vi "UHR-Fleezers Control (host) - 10.6.vi"() -> ()   [LabVIEW 2011] (continued)
        n2246 = call <vilib>:"Mean.vi"("X"=w3459) -> ("mean"=w3450:dbl)  [unwired: 1 out]
        n2247 = Subtract(x=w3554, y=w3546) -> (x-y=w3488:u64)
        n2248 = call <vilib>:"Mean.vi"("X"=w3544) -> ("mean"=w3485:dbl)  [unwired: 1 out]
        n2249 = Initialize Array(1.0 ("element"), w3453) -> (w3449:dbl[])
        n2250 = Initialize Array(1.0 ("element"), w3488) -> (w3479:dbl[])
        n2251 = Multiply(x=w3449, y=w3450) -> (x*y=w3451:dbl[])
        n2252 = Multiply(x=w3479, y=w3481) -> (x*y=w3482:dbl[])
        n2253 = Multiply(x=w3479, y=w3483) -> (x*y=w3484:dbl[])
        n2254 = Multiply(x=w3479, y=w3478) -> (x*y=w3480:dbl[])
        n2255 = Multiply(x=w3479, y=w3485) -> (x*y=w3486:dbl[])
        n2256 = Build Array (concatenate)(w3494, w3480) -> (w3548:dbl[])
        n2257 = Build Array (concatenate)(w3496, w3484) -> (w3552:dbl[])
        n2258 = Build Array (concatenate)(w3495, w3482) -> (w3551:dbl[])
        n2259 = Build Array (concatenate)(w3459, w3451) -> (w3461:dbl[])
        n2260 = Build Array (concatenate)(w3544, w3486) -> (w3553:dbl[])
        n2261 = Reshape Array(w3548, w3432, w3431) -> (w3514:dbl[][])
        n2262 = Reshape Array(w3461, w3432, w3431) -> (w3457:dbl[][])
        n2263 = Reshape Array(w3552, w3432, w3431) -> (w3506:dbl[][])
        n2264 = Reshape Array(w3551, w3432, w3431) -> (w3521:dbl[][])
        n2265 = Reshape Array(w3553, w3432, w3431) -> (w3531:dbl[][])
        n2266 = Array Subset(array=w3521, index (col)=0 ("index"), length (col)=w3446) -> (w3526:dbl[][])  [unwired: 2 in]
        n2267 = Array Subset(array=w3521, index (col)=w3446) -> (w3524:dbl[][])  [unwired: 3 in]
        n2268 = Array Subset(array=w3506, index (col)=0 ("index"), length (col)=w3446) -> (w3512:dbl[][])  [unwired: 2 in]
        n2269 = Array Subset(array=w3506, index (col)=w3446) -> (w3510:dbl[][])  [unwired: 3 in]
        n2270 = Array Subset(array=w3457, index (col)=0 ("index"), length (col)=w3446) -> (w3456:dbl[][])  [unwired: 2 in]
        n2271 = Array Subset(array=w3457, index (col)=w3446) -> (w3454:dbl[][])  [unwired: 3 in]
        n2272 = Array Subset(array=w3531, index (col)=0 ("index"), length (col)=w3446) -> (w3530:dbl[][])  [unwired: 2 in]
        n2273 = Array Subset(array=w3531, index (col)=w3446) -> (w3528:dbl[][])  [unwired: 3 in]
        n2274 = Array Subset(array=w3514, index (col)=0 ("index"), length (col)=w3446) -> (w3519:dbl[][])  [unwired: 2 in]
        n2275 = Array Subset(array=w3514, index (col)=w3446) -> (w3517:dbl[][])  [unwired: 3 in]
        n2276 = for {
          tunnel: w3526 -> [w3568] mode=indexing
          tunnel: [w3567] -> w3525 mode=indexing
          workers-P: _ -> [_]
          n2277 = Reverse 1D Array(array=w3568) -> (reversed array=w3567:dbl[])
        }
        n2278 = for {
          tunnel: w3512 -> [w3564] mode=indexing
          tunnel: [w3563] -> w3511 mode=indexing
          workers-P: _ -> [_]
          n2279 = Reverse 1D Array(array=w3564) -> (reversed array=w3563:dbl[])
        }
        n2280 = for {
          tunnel: w3456 -> [w3562] mode=indexing
          tunnel: [w3561] -> w3455 mode=indexing
          workers-P: _ -> [_]
          n2281 = Reverse 1D Array(array=w3562) -> (reversed array=w3561:dbl[])
        }
        n2282 = for {
          tunnel: w3530 -> [w3570] mode=indexing
          tunnel: [w3569] -> w3529 mode=indexing
          workers-P: _ -> [_]
          n2283 = Reverse 1D Array(array=w3570) -> (reversed array=w3569:dbl[])
        }
        n2284 = for {
          tunnel: w3519 -> [w3566] mode=indexing
          tunnel: [w3565] -> w3518 mode=indexing
          workers-P: _ -> [_]
          n2285 = Reverse 1D Array(array=w3566) -> (reversed array=w3565:dbl[])
        }
        n2286 = Index Array(array=w3531, index (row)=0) -> (element=→"Waveform Graph":dbl[])  [unwired: 1 in]
        n2287 = Add(x=w3525, y=w3524) -> (x+y=w3523:dbl[][])
        n2288 = Add(x=w3511, y=w3510) -> (x+y=w3509:dbl[][])
        n2289 = Add(x=w3455, y=w3454) -> (x+y=w3439:dbl[][])
        n2290 = Add(x=w3529, y=w3528) -> (x+y=w3503:dbl[][])
        n2291 = Add(x=w3518, y=w3517) -> (x+y=w3516:dbl[][])
        n2292 = Divide(x=w3509, y=2) -> (x/y=w3507:dbl[][])
        n2293 = Divide(x=w3523, y=2) -> (x/y=w3468:dbl[][])
        n2294 = Divide(x=w3516, y=2) -> (x/y=w3470:dbl[][])
        n2295 = To Single Precision Float(number=w3503) -> (single precision float=w3502:sgl[][])
        n2296 = Transpose 2D Array(2D array=w3507) -> (transposed array=→"Data map":dbl[][])
        n2297 = To Single Precision Float(number=w3439) -> (single precision float=w3443:sgl[][])
        n2298 = To Single Precision Float(number=w3468) -> (single precision float=w3474:sgl[][])
        n2299 = To Single Precision Float(number=w3470) -> (single precision float=w3471:sgl[][])
        n2300 = call "IMAQ ArrayToImage"("Image Pixels (Float)"=w3502, "Image"=w3436) -> ("Image Out"=w3505:T2)  [unwired: 8 in, 1 out]
        n2301 = call "IMAQ ArrayToImage"("Image Pixels (Float)"=w3443, "Image"=w3435) -> ("Image Out"=w3445:T2)  [unwired: 8 in, 1 out]
        n2302 = call "IMAQ ArrayToImage"("Image Pixels (Float)"=w3474, "Image"=w3434) -> ("Image Out"=w3476:T2)  [unwired: 8 in, 1 out]
        n2303 = call "IMAQ ArrayToImage"("Image Pixels (Float)"=w3471, "Image"=w3433) -> ("Image Out"=w3473:T2)  [unwired: 8 in, 1 out]
        n2304 = call "IMAQ Symmetry"("Type of Symmetry"=w3504, "Image Src"=w3505) -> ("Image Dst Out"=w3500:T2)  [unwired: 3 in, 1 out]
        n2305 = call "IMAQ Symmetry"("Type of Symmetry"=w3444, "Image Src"=w3445) -> ("Image Dst Out"=w3441:T2)  [unwired: 3 in, 1 out]
        n2306 = call "IMAQ Symmetry"("Type of Symmetry"=w3475, "Image Src"=w3476) -> ("Image Dst Out"=→"Detection Laser X":T2)  [unwired: 3 in, 1 out]
        n2307 = call "IMAQ Symmetry"("Type of Symmetry"=w3472, "Image Src"=w3473) -> ("Image Dst Out"=→"Detection Laser Y":T2)  [unwired: 3 in, 1 out]
        n2308 = call "IMAQ Set Simple Calibration"("Calibration Axis Info"=T35 {"Origin Pixel"={"X"=0.0, "Y"=0.0}, "Angle Relative to Horizontal (deg)"=0.0, "Axis Reference"=0}, "Grid Descriptor"=T36 {"X Step"=0.3, "Y Step"=0.3, "Unit"=enum."Undefined"}, "Image"=w3500) -> ("Calibrated Image"=→"APD 1":T2)  [unwired: 7 in, 1 out]
        n2309 = call "IMAQ Set Simple Calibration"("Calibration Axis Info"=T35 {"Origin Pixel"={"X"=0.0, "Y"=0.0}, "Angle Relative to Horizontal (deg)"=0.0, "Axis Reference"=0}, "Grid Descriptor"=T36 {"X Step"=0.3, "Y Step"=0.3, "Unit"=enum."Undefined"}, "Image"=w3441) -> ("Calibrated Image"=→"APD 2":T2)  [unwired: 7 in, 1 out]
      }
    }
    n2310 = Subtract(x=w2945, y="APD 2 Offset") -> (x-y=w2942:waveform(dbl))
    n2311 = Subtract(x=w2947, y="APD 1 Offset") -> (x-y=w2943:waveform(dbl))
    n2312 = Index Array(array=w2962, index=3) -> (element=w3022:waveform(dbl))
    n2313 = Index Array(array=w2962, index=6) -> (element=w3019:waveform(dbl))
    n2314 = Build Array(w2943, w2942) -> (→"APD Chart":waveform(dbl)[])
    n2315 = Array Size(array=w3013) -> (size(s)=w3066:i32)
    n2316 = call <vilib>:"Std Deviation and Variance.vi"("X"=w2955) -> ("standard deviation"=w2954:dbl)  [unwired: 1 in, 2 out]
    n2317 = Add Array Elements(numeric array=w2955) -> (sum=w2957:u32)
    n2318 = Add Array Elements(numeric array=w3013) -> (sum=w3076:u32)
    n2319 = call <vilib>:"Std Deviation and Variance.vi"("X"=w3013) -> ("standard deviation"=w3012:dbl)  [unwired: 1 in, 2 out]
    n2320 = Divide(x="T1 offset_x (mV)", y=1000.0) -> (x/y=w3023:dbl)
    n2321 = Divide(x=w2954, y=w2953) -> (x/y=w2950:dbl)
    "Rate sigma (Hz) 2" <- w2950
    n2322 = Multiply(x=w2953, y=w3066) -> (x*y=w2956:dbl)
    "Int. Time (s)" <- w2956
    n2323 = Divide(x=w2957, y=w2956) -> (x/y=w2951:dbl)
    "APD 2 Rate (Hz)" <- w2951
    n2324 = Divide(x=w3076, y=w2956) -> (x/y=w3010:dbl)
    "APD 1 Rate (Hz)" <- w3010
    n2325 = Divide(x=w3012, y=w2953) -> (x/y=w3011:dbl)
    "Rate sigma (Hz)" <- w3011
    n2326 = Divide(x=w2950, y=w2951) -> (x/y=→"Sigma/Mean 2":dbl)
    n2327 = Divide(x=w3011, y=w3010) -> (x/y=→"Sigma/Mean":dbl)
    n2328 = feedback-in #22("Calibration") -> ()
    n2329 = feedback #22(u16 1 ("Calibration")) -> (w3043:u16)
    n2330 = Divide(x="T2 offset_x (mV)", y=1000.0) -> (x/y=w3021:dbl)
    n2331 = case shown="0, Default" "Calibration" {
      tunnel: "T1 alpha_x (nm/V)" -> [_ w3399 w3420]
      tunnel: "T1 kappa_x (pN/nm)" -> [_ _ w3410]
      tunnel: "T2 alpha_x (nm/V)" -> [_ w3398 w3418]
      tunnel: "T2 kappa_x (pN/nm)" -> [_ _ w3411]
      tunnel: w3022 -> [w3381 w3396 w3416]
      tunnel: w3019 -> [w3380 w3394 w3414]
      tunnel: [w3381 w3393 w3413] -> w3052
      tunnel: [w3380 w3392 w3412] -> w3051
      tunnel: ["T1 X (V)" ("Label.Text") "T1 X (nm)" ("Label.Text") "T1 X (pN)" ("Label.Text")] -> w3040
      tunnel: ["T2 X (V)" ("Label.Text") "T2 X (nm)" ("Label.Text") "T2 X (pN)" ("Label.Text")] -> w3039
      tunnel: ["Position (V)" ("Label.Text") "Position (nm)" ("Label.Text") "Force (pN)" ("Label.Text")] -> w3041
      tunnel: w3021 -> [_ w3384 w3403]
      tunnel: w3023 -> [_ w3387 w3405]
      tunnel: ["Mean (V)" ("Label.Text") "Mean (nm)" ("Label.Text") "Mean (pN)" ("Label.Text")] -> w3036
      tunnel: ["Difference (V)" ("Label.Text") "Difference (nm)" ("Label.Text") "Difference (pN)" ("Label.Text")] -> w2970
      frame 0, Default {
      }
      frame 1 {
        n2332 = Unbundle By Name(w3396) -> ("Y"=w3400:dbl[])
        n2333 = Unbundle By Name(w3394) -> ("Y"=w3385:dbl[])
        n2334 = Subtract(x=w3400, y=w3387) -> (x-y=w3388:dbl[])
        n2335 = Subtract(x=w3385, y=w3384) -> (x-y=w3386:dbl[])
        n2336 = Multiply(x=w3386, y=w3398) -> (x*y=w3395:dbl[])
        n2337 = Multiply(x=w3399, y=w3388) -> (x*y=w3397:dbl[])
        n2338 = Bundle By Name(cluster=w3394, "Y"=w3395) -> (w3392:waveform(dbl))
        n2339 = Bundle By Name(cluster=w3396, "Y"=w3397) -> (w3393:waveform(dbl))
      }
      frame 2 {
        n2340 = Unbundle By Name(w3416) -> ("Y"=w3421:dbl[])
        n2341 = Unbundle By Name(w3414) -> ("Y"=w3419:dbl[])
        n2342 = Subtract(x=w3419, y=w3403) -> (x-y=w3404:dbl[])
        n2343 = Subtract(x=w3421, y=w3405) -> (x-y=w3406:dbl[])
        n2344 = Compound Arithmetic op=MULTIPLY(w3404, w3418, w3411) -> (w3415:dbl[])
        n2345 = Compound Arithmetic op=MULTIPLY(w3410, w3420, w3406) -> (w3417:dbl[])
        n2346 = Bundle By Name(cluster=w3414, "Y"=w3415) -> (w3412:waveform(dbl))
        n2347 = Bundle By Name(cluster=w3416, "Y"=w3417) -> (w3413:waveform(dbl))
      }
    }
    n2348 = Not Equal?(x=w3043, y="Calibration") -> (x != y?=w3000:bool)
    n2349 = case shown="True" w3000 {
      tunnel: w3041 -> [_ w3374]
      tunnel: w3040 -> [_ w3373]
      tunnel: w3039 -> [_ w3372]
      tunnel: w3036 -> [_ w3371]
      tunnel: w2970 -> [_ w3370]
      frame False {
      }
      frame True {
        n2350 = property on="Force" class="WFChart (strict)"("YScale.NameLbl.Text"=w3374) -> ()  [unwired: 2 in, 2 out]
        n2351 = property on="T2 X" class="DigNum (strict)"("Caption.Text"=w3372) -> ()  [unwired: 2 in, 2 out]
        n2352 = property on="T1 X" class="DigNum (strict)"("Caption.Text"=w3373) -> ()  [unwired: 2 in, 2 out]
        n2353 = property on="Mean" class="DigNum (strict)"("Caption.Text"=w3371) -> ()  [unwired: 2 in, 2 out]
        n2354 = property on="Difference" class="DigNum (strict)"("Caption.Text"=w3370) -> ()  [unwired: 2 in, 2 out]
      }
    }
    n2355 = Unbundle By Name(w3022) -> ("Y"=w3025:dbl[])
    n2356 = Unbundle By Name(w3019) -> ("Y"=w3028:dbl[])
    n2357 = Subtract(x=w3025, y=w3023) -> (x-y=w3026:dbl[])
    n2358 = Subtract(x=w3028, y=w3021) -> (x-y=w3027:dbl[])
    n2359 = Multiply(x=w3027, y="T2 alpha_x (nm/V)") -> (x*y=w2811:dbl[])
    n2360 = Multiply(x="T1 alpha_x (nm/V)", y=w3026) -> (x*y=w2812:dbl[])
    n2361 = Not(x="Trap Trig. Fl.") -> (.not. x?=w2849:bool)
    n2362 = Multiply(x=w3051, y=-1.0) -> (x*y=w3030:waveform(dbl))
    n2363 = Subtract(x=w2812, y=w2811) -> (x-y=w3018:dbl[])
    n2364 = Unbundle By Name(w3051) -> ("Y"=w2989:dbl[])
    n2365 = Unbundle By Name(w3052) -> ("Y"=w2813:dbl[])
    n2366 = Negate(x=w3018) -> (-x=w2809:dbl[])
    n2367 = Build Array(w3052, w3030) -> (→"Force":waveform(dbl)[])
    n2368 = Subtract(x=w2809, y="Offset (nm)") -> (x-y=w2987:dbl[])
    n2369 = case shown="True" "Read Lateness and Rel Phase" {
      tunnel: w2829 -> [w3347 w3369]
      tunnel: w2828 -> [w3348 w3368]
      tunnel: [w3347 w3367] -> w3016
      tunnel: [w3348 w3366] -> w3015
      frame False {
      }
      frame True {
        n2370 = xnode "Read/Write Control"("FPGA VI Reference In"=w3369, "error in"=w3368) -> ("FPGA VI Reference Out"=w3367:T19, "error out"=w3366:errorcluster, "GI Relative phase"=→"GI relative phase":i16, "Relative phase"=→"Relative phase (AI1)":i16, "AI Late Counter"=→"Late Counter (AI1)":u16, "GI Late Counter"=→"GI Late Counter":u16, "MCL Late Counter"=→"MCL Late Counter":u16, "MCL Relative Phase"=→"Relative Phase (MCL)":i16, "APD Acq Relative Phase"=→"APD Acq Relative Phase":i16, "APD 1 Gate Relative Phase"=→"APD 1 Gate Relative Phase":i16, "APD 2 Gate Relative Phase"=→"APD 2 Gate Relative Phase":i16, "APD Acq Late Counter"=→"APD Acq Late Counter":u16, "APD 1 Gate Late Counter"=→"APD 1 Gate Late Counter":u16, "APD 2 Gate Late Counter"=→"APD 2 Gate Late Counter":u16, "Green FB Relative Phase"=→"Relative phase (Green FB)":i16, "GI Relative phase 2"=→"GI relative phase 2":i16, "GI Late Counter 2"=→"GI Late Counter 2":u16, "Trap Pos FIFO Timeout"=→"Trap Pos FIFO Timeout":u16, "Trap AI FIFO Timeout"=→"Trap AI FIFO Timeout":u16)
      }
    }
    n2371 = call <vilib>:"Mean.vi"("X"=w2989) -> ("mean"=w2815:dbl)  [unwired: 1 out]
    "T2 X" <- w2815
    n2372 = Negate(x=w2989) -> (-x=w2990:dbl[])
    n2373 = call <vilib>:"Mean.vi"("X"=w2813) -> ("mean"=w2816:dbl)  [unwired: 1 out]
    "T1 X" <- w2816
    n2374 = Negate(x=w2815) -> (-x=w2814:dbl)
    n2375 = Bundle By Name(cluster=w3022, "Y"=w2987) -> (w2961:waveform(dbl))
    "Bead Separation" <- w2961
    n2376 = Add(x=w2813, y=w2990) -> (x+y=w2991:dbl[])
    n2377 = Add(x=w2816, y=w2814) -> (x+y=w3038:dbl)
    n2378 = Subtract(x=w2816, y=w2814) -> (x-y=→"Difference":dbl)
    n2379 = Divide(x=w2991, y=2.0) -> (x/y=→"Vec Mean of T1 T2":dbl[])
    n2380 = Divide(x=w3038, y=2.0) -> (x/y=w2993:dbl)
    "Mean" <- w2993
    n2381 = feedback-in #23("Trap Trig. Fl.") -> ()
    n2382 = feedback #23("Trap Trig. Fl.") -> (w2847:bool)
    n2383 = And(x=w2849, y=w2847) -> (x .and. y?=w2848:bool)
    n2384 = case "If have just turned off triggering" shown="True" w2848 {
      tunnel: w2829 -> [_ w3182]
      tunnel: w2828 -> [_ w3181]
      frame False {
      }
      frame True {
        w3180 = FALSE ("FPGA Trap Trig")
        n2385 = xnode "Read/Write Control"("FPGA VI Reference In"=w3182, "error in"=w3181, "FPGA Trap Trig"=w3180) -> ("FPGA VI Reference Out"=w3179:T19, "error out"=w3178:errorcluster)
        n2386 = xnode "Read/Write Control"("FPGA VI Reference In"=w3179, "error in"=w3178, "TTrig?"=w3180) -> ()  [unwired: 2 out]
        n2387 = local write "Initializing"(FALSE ("Initializing")) -> ()
        n2388 = local write "Triggered"(FALSE ("Triggered")) -> ()
        n2389 = local write "Waiting"(FALSE ("Waiting")) -> ()
      }
    }
    n2390 = Not(x=w2847) -> (.not. x?=w2860:bool)
    n2391 = And(x="Trap Trig. Fl.", y=w2860) -> (x .and. y?=w2857:bool)
    n2392 = local read "Tether"() -> (w2994:bool)
    n2393 = Or(x=w2857, y="Reinitialize") -> (x .or. y?=w2843:bool)
    n2394 = feedback #24(w2853) -> (w2858:string)
    n2395 = Select(t=w2853, s=w2857, f=w2858) -> (s? t:f=w2852:string)
    n2396 = Select(t=w2853, s="Reinitialize", f=w2852) -> (s? t:f=w2851:string)
    n2397 = feedback #25(0) -> (w2855:i32)
    n2398 = feedback #26(w2987) -> (w2986:dbl[])
    n2399 = Build Array (concatenate)(w2987, w2986) -> (w2810:dbl[])
    n2400 = case "For determining if there is a tether still" shown="True" w2994 {
      tunnel: w2993 -> [_ w3306]
      frame False {
      }
      frame True {
        n2401 = Greater?(x="Lost Tether Alarm Threshold (pN)", y=w3306) -> (0:w3304:bool)
        n2402 = case shown="True" w3304 {
          frame False {
          }
          frame True {
            w3307 = FALSE ("Value (Signaling)")
            n2403 = flat-sequence {
              frame #0 {
                # "stop only if saving"
                n2404 = local read "Saving..."() -> (w3319:bool)
                n2405 = And(x=w3319, y="TA Cancel Save?") -> (x .and. y?=w3318:bool)
                n2406 = local write "Stop Saving"(w3318) -> ()
              }
              frame #1 {
                n2407 = case shown="True" "TA Green Off?" {
                  frame False {
                  }
                  frame True {
                    w3322 = FALSE ("Fl. Triggered...")
                    n2408 = local write "Fl. Triggered..."(w3322) -> ()
                    n2409 = property on="Green Laser ON/Interlacing" class="Bool (strict)"("Val(Sgnl)"=w3322) -> ()  [unwired: 2 in, 2 out]
                  }
                }
              }
            }
            n2410 = local read "Time tether formed"() -> (w3313:timestamp)
            n2411 = Get Date/Time In Seconds() -> (seconds since 1Jan1904=w3314:timestamp)
            n2412 = Subtract(x=w3314, y=w3313) -> (x-y=w3312:dbl)
            n2413 = Number To Decimal String(number=w3312) -> (decimal integer string=w3309:string)  [unwired: 1 out]
            n2414 = local read "Messages"() -> (w3316:string)
            n2415 = call <vilib>:"Beep.vi"() -> ()  [unwired: 3 in, 9 out]
            n2416 = Concatenate Strings("Lost tether (" ("Message to add"), w3309, " s)." ("string")) -> (w3311:string)
            n2417 = local write "Tether"(FALSE ("Tether")) -> ()
            n2418 = call "Update messages.vi"("Message to add"=w3311, "Old message string"=w3316) -> ("New message string"=w3315:string)
            n2419 = local write "Messages"(w3315) -> ()
            n2420 = local write "Dip for Protein"(w3307) -> ()
            n2421 = property on="Trap Pos. FB ON" class="Bool (strict)"("Val(Sgnl)"=w3307) -> ()  [unwired: 2 in, 2 out]
            n2422 = property on="Trap Trig. Fl." class="Bool (strict)"("Val(Sgnl)"=w3307) -> ()  [unwired: 2 in, 2 out]
          }
        }
      }
    }
    n2423 = case "For triggering actions based on the trap position (e.g., turning the excitation laser on if trap under feedback moves so far)" shown="True" "Trap Trig. Fl." {
      tunnel: w2838 -> [_ w3195]
      tunnel: w2851 -> [_ w3194]
      tunnel: ["" ("t") w3193] -> w2859
      tunnel: w2843 -> [_ w3192]
      tunnel: [0 ("t") w3191] -> w2856
      tunnel: w2855 -> [_ w3190]
      tunnel: w2829 -> [_ w3189]
      tunnel: w2828 -> [_ w3188]
      frame False {
      }
      frame True {
        n2424 = case shown="\"Wait for trigger\"" w3194 {
          tunnel: w3195 -> [w3212 _ _ w3260]
          tunnel: [w3209 w3241 "" ("t") w3263] -> w3193
          tunnel: w3192 -> [_ _ _ w3251]
          tunnel: [w3208 w3238 0 ("t") w3252] -> w3191
          tunnel: w3190 -> [_ w3240 _ w3258]
          tunnel: w3189 -> [w3197 w3235 _ w3254]
          tunnel: w3188 -> [w3196 w3234 _ w3253]
          frame "Wait for trigger" {
            n2425 = local read "Trap Trig. (FPGA)"() -> (w3200:bool)
            n2426 = Subtract(x=w3212, y="Mean T1 Position\nto compare (nm)") -> (x-y=w3205:dbl[])
            n2427 = call <vilib>:"Std Deviation and Variance.vi"("X"=w3205) -> ("mean"=→"mean":dbl, "standard deviation"=→"standard\ndeviation":dbl)  [unwired: 1 in, 1 out]
            n2428 = Array Max & Min(array=w3205) -> (max value=→"max value":dbl, min value=→"min value":dbl)  [unwired: 2 out]
            n2429 = Greater?(x=w3205, y="Threshold (nm)") -> (0:w3215:bool[])
            n2430 = case shown="True" w3200 {
              tunnel: w3197 -> [_ w3221]
              tunnel: w3196 -> [_ w3220]
              tunnel: [FALSE ("TTrig?") w3219] -> w3203
              frame False {
              }
              frame True {
                n2431 = xnode "Read/Write Control"("FPGA VI Reference In"=w3221, "error in"=w3220) -> ("TTrig?"=w3219:bool)  [unwired: 2 out]
              }
            }
            n2432 = Or Array Elements(Boolean array=w3215) -> (logical OR=w3202:bool)
            n2433 = Select(t=w3203, s=w3200, f=w3202) -> (s? t:f=w3201:bool)
            n2434 = Not(x=w3200) -> (.not. x?=w3199:bool)
            n2435 = And(x=w3201, y=w3199) -> (x .and. y?=w3198:bool)
            n2436 = Select(t="Triggered", s=w3201, f="Wait for trigger") -> (s? t:f=w3209:string)
            n2437 = case shown="True" w3201 {
              tunnel: [0 0] -> w3208
              tunnel: w3197 -> [_ w3226]
              tunnel: w3196 -> [_ w3225]
              frame False {
                "Waiting" <- TRUE ("Waiting")
              }
              frame True {
                n2438 = xnode "Read/Write Control"("FPGA VI Reference In"=w3226, "error in"=w3225, "TTrig?"=FALSE) -> ()  [unwired: 2 out]
                n2439 = local read "Messages"() -> (w3229:string)
                n2440 = call <vilib>:"Beep.vi"() -> ()  [unwired: 12 in]
                n2441 = call "Update messages.vi"("Message to add"="Unwinding trigger.", "Old message string"=w3229) -> ("New message string"=w3230:string)
                n2442 = local write "Messages"(w3230) -> ()
                n2443 = local write "Waiting"(FALSE ("Waiting")) -> ()
                "Triggered" <- TRUE ("Triggered")
              }
            }
            n2444 = case "Only need to turn on laser if host triggered" shown="True" w3198 {
              frame False {
              }
              frame True {
                n2445 = property on="Green Laser ON/Interlacing" class="Bool (strict)"("Val(Sgnl)"=TRUE ("Value (Signaling)")) -> ()  [unwired: 2 in, 2 out]
              }
            }
          }
          frame "Triggered" {
            n2446 = local read "Trap Trig. (FPGA)"() -> (w3237:bool)
            n2447 = Increment(x=w3240) -> (x+1=w3238:i32)
            n2448 = Greater Or Equal?(x=w3238, y="Fl. ON time (n)") -> (x >= y?=w3236:bool)
            n2449 = Select(t="Wait for trigger", s=w3236, f="Triggered" ("t")) -> (s? t:f=w3241:string)
            n2450 = And(x=w3236, y=w3237) -> (x .and. y?=w3233:bool)
            n2451 = case shown="True" w3233 {
              tunnel: w3235 -> [_ w3245]
              tunnel: w3234 -> [_ w3244]
              frame False {
              }
              frame True {
                n2452 = xnode "Read/Write Control"("FPGA VI Reference In"=w3245, "error in"=w3244, "FPGA Trap Trig"=TRUE) -> ()  [unwired: 2 out]
              }
            }
            n2453 = case shown="True" w3236 {
              frame False {
              }
              frame True {
                w3247 = FALSE ("Value (Signaling)")
                n2454 = local write "Triggered"(w3247) -> ()
                n2455 = local write "Waiting"(TRUE ("Waiting")) -> ()
                n2456 = property on="Green Laser ON/Interlacing" class="Bool (strict)"("Val(Sgnl)"=w3247) -> ()  [unwired: 2 in, 2 out]
              }
            }
          }
          frame "Do nothing" {
          }
          frame "Initialize", Default {
            n2457 = Increment(x=w3258) -> (x+1=w3262:i32)
            n2458 = Select(t=1, s=w3251, f=w3262) -> (s? t:f=w3252:i32)
            n2459 = feedback #27(w3260) -> (w3266:dbl[])
            n2460 = Build Array (concatenate)(w3260, w3266) -> (w3259:dbl[])
            n2461 = Greater Or Equal?(x=w3252, y="Wait to get offset (n)") -> (x >= y?=w3255:bool)
            n2462 = Select(t=w3260, s=w3251, f=w3259) -> (s? t:f=w3261:dbl[])
            n2463 = feedback-in #27(w3261) -> ()
            n2464 = call <vilib>:"Mean.vi"("X"=w3261) -> ("mean"=w3256:dbl)  [unwired: 1 out]
            n2465 = local write "Mean T1 Position\nto compare (nm)"(w3256) -> ()
            n2466 = case shown="True" w3251 {
              tunnel: w3254 -> [_ w3272]
              tunnel: w3253 -> [_ w3271]
              frame False {
              }
              frame True {
                w3268 = FALSE ("FPGA Trap Trig")
                n2467 = xnode "Read/Write Control"("FPGA VI Reference In"=w3272, "error in"=w3271, "FPGA Trap Trig"=w3268) -> ("FPGA VI Reference Out"=w3270:T19, "error out"=w3269:errorcluster)
                n2468 = xnode "Read/Write Control"("FPGA VI Reference In"=w3270, "error in"=w3269, "TTrig?"=w3268) -> ()  [unwired: 2 out]
              }
            }
            n2469 = Select(t="Wait for trigger", s=w3255, f="Initialize") -> (s? t:f=w3263:string)
            n2470 = case shown="True" w3255 {
              tunnel: w3256 -> [_ w3275]
              tunnel: w3254 -> [_ w3284]
              tunnel: w3253 -> [_ w3283]
              frame False {
                n2471 = local write "Waiting"(FALSE ("Waiting")) -> ()
                "Initializing" <- TRUE ("Initializing")
              }
              frame True {
                n2472 = local read "Threshold (nm)"() -> (w3287:dbl)
                n2473 = local read "AOM X Cal (nm/MHz)"() -> (w3286:dbl)
                n2474 = Add(x=w3275, y=w3287) -> (x+y=w3288:dbl)
                n2475 = Divide(x=w3288, y=w3286) -> (x/y=w3285:dbl)
                n2476 = call "IR AOM freq to word.vi"("Frequency In (MHz)"=w3285) -> ("Frequency Word Out (double)"=w3282:dbl)
                n2477 = local write "Initializing"(FALSE ("Initializing")) -> ()
                n2478 = local write "Waiting"(TRUE ("Waiting")) -> ()
                n2479 = To Quad Integer(1:w3282) -> (0:w3281:i64)
                n2480 = xnode "Read/Write Control"("FPGA VI Reference In"=w3284, "error in"=w3283, "FPGA TTrig Thresh"=w3281) -> ("FPGA VI Reference Out"=w3278:T19, "error out"=w3277:errorcluster)
                n2481 = xnode "Read/Write Control"("FPGA VI Reference In"=w3278, "error in"=w3277, "FPGA Trap Trig"=TRUE) -> ()  [unwired: 2 out]
              }
            }
          }
        }
      }
    }
    n2482 = feedback-in #24(w2859) -> ()
    n2483 = feedback-in #25(w2856) -> ()
    n2484 = Split 1D Array(array=w2810, index=w2873) -> (first subarray=w2983:dbl[])  [unwired: 1 out]
    n2485 = feedback-in #26(w2983) -> ()
    n2486 = call <vilib>:"Mean.vi"("X"=w2983) -> ("mean"=w2982:dbl)  [unwired: 1 out]
    "Bead Mean (nm)" <- w2982
    n2487 = Subtract(x=w2983, y=w2982) -> (x-y=w2981:dbl[])
    n2488 = Square(x=w2981) -> (x^2=w2980:dbl[])
    n2489 = call <vilib>:"Mean.vi"("X"=w2980) -> ("mean"=w2979:dbl)  [unwired: 1 out]
    n2490 = Square Root(x=w2979) -> (sqrt(x)=w2978:dbl)
    n2491 = Multiply(x=10.0, y=w2978) -> (x*y=→"RMS (Ang)":dbl)
    n2492 = xnode "Read/Write Control"("FPGA VI Reference In"=w3016, "error in"=w3015) -> ("FPGA VI Reference Out"=w2841:T19, "error out"=w2840:errorcluster, "AI2 Y Sum Set 1"=w3122:i16, "AI2 Y Sum Set 2"=w3121:i16, "AI1 X Set 1"=w2905:fxp<+/-,16,1>, "AI1 X Set 2"=w2904:fxp<+/-,16,1>, "Trap Pos FB Int Signal"=→"Trap Pos FB Int Signal":fxp<+/-,24,9>, "Trap Pos FB Int-Norm Signal"=→"Trap Pos FB Int-Norm Signal":fxp<+/-,16,1>, "Trap Pos FB Action"=w2898:i64, "Scanning"=→"AOD Scanning":bool, "Scan I"=→"AOD Scan I":u64, "Scanning MCL"=w3124:bool, "Scan I (MCL)"=→"MCL Scan I":u64, "Green FB Signals"=w3061:T46, "TTrig Sig"=w2827:i64, "TTrig Fin Thresh"=w2823:i64)
    "MCL Scanning" <- w3124
    "Trap Pos FB Action" <- w2898
    n2493 = local read "FB Trig Integrate"() -> (w2821:u32)
    n2494 = Divide(x=w2827, y=w2821) -> (x/y=w2820:dbl)
    "TTrig Sig (Int)" <- w2820
    n2495 = Divide(x=w2823, y=w2821) -> (x/y=w2818:dbl)
    "TTrig Fin Thresh (Int)" <- w2818
    n2496 = local read "AOM X Cal (nm/MHz)"() -> (w2826:dbl)
    n2497 = local read "AI2 (V)"() -> (w3123:cluster{"Set 1":dbl, "Set 2":dbl})
    n2498 = Bundle By Name(cluster=w3123, "Set 1"=w3122, "Set 2"=w3121) -> (w3119:cluster{"Set 1":dbl, "Set 2":dbl})
    n2499 = Divide(x=w2898, y=327.67) -> (x/y=→"Action (%)":dbl)
    n2500 = local read "Trap X (AI1)"() -> (w2918:T10)
    n2501 = call "IR AOM word double to freq.vi"("Frequency Word In (double)"=w2818) -> ("Frequency Out (MHz)"=w2817:dbl)
    n2502 = call "IR AOM word double to freq.vi"("Frequency Word In (double)"=w2820) -> ("Frequency Out (MHz)"=w2819:dbl)
    n2503 = Divide(x=w3119, y=3276.7) -> (x/y=w3118:cluster{"Set 1":dbl, "Set 2":dbl})
    n2504 = Multiply(x=w2819, y=w2826) -> (x*y=w2825:dbl)
    "TTrig Sig (nm)" <- w2825
    n2505 = Multiply(x=w2817, y=w2826) -> (x*y=w2824:dbl)
    "TTrig Fin Thresh (nm)" <- w2824
    n2506 = local write "AI2 (V)"(w3118) -> ()
    n2507 = Bundle(cluster=w2918, "Trap 1"=w2905, "Trap 2"=w2904) -> (→"Trap X (AI1)":T10)
    n2508 = Bundle(w2825, w2824) -> (→"TTrig":cluster{dbl, dbl})  [unwired: 1 in]
    n2509 = Divide(x=w3061, y=3276.7) -> (x/y=w3057:T47)
    n2510 = Unbundle By Name(w3057) -> ("Green FB Ch 0"=w3060:dbl, "Green FB Ch 1"=w3059:dbl, "Green FB Ch 2"=w3058:dbl)
    n2511 = Divide(x=w3060, y=w3058) -> (x/y=w3056:dbl)
    n2512 = Divide(x=w3059, y=w3058) -> (x/y=w3055:dbl)
    n2513 = flat-sequence "To save data" {
      tunnel: [w4143] -> w3142
      tunnel: [w4144] -> w3141
      tunnel: w3092 -> [w4137]
      tunnel: w2846 -> [w4141]
      tunnel: ["Save Calibration"] -> w3115
      tunnel: w3112 -> [w4140]
      tunnel: [w4133] -> w3111
      tunnel: [w4130] -> w3110
      tunnel: [w4127] -> w3109
      tunnel: w3091 -> [w4129]
      tunnel: w2998 -> [w4123]
      tunnel: [w4123] -> w2997
      tunnel: ["Start Saving"] -> w2963
      tunnel: [w4117] -> w2886
      tunnel: [w4116] -> w2885
      tunnel: w3142 -> [w4378]
      tunnel: w3141 -> [w4377]
      tunnel: w2887 -> [w4376]
      tunnel: w3115 -> [w4375]
      tunnel: w3111 -> [w4373]
      tunnel: w3110 -> [w4372]
      tunnel: w3109 -> [w4371]
      tunnel: w2972 -> [w4370]
      tunnel: w3008 -> [w4369]
      tunnel: w2997 -> [w4368]
      tunnel: w2963 -> [w4367]
      tunnel: w2961 -> [w4366]
      tunnel: w2937 -> [w4365]
      tunnel: w2886 -> [w4364]
      tunnel: w2885 -> [w4363]
      tunnel: w2884 -> [w4362]
      frame #0 {
        n2514 = Or(x="Save N Sets", y="Start Saving") -> (x .or. y?=w4124:bool)
        n2515 = To Double Precision Float(number=w4140) -> (double precision float=w4134:dbl)
        n2516 = Build Array(w4124, "Save Calibration", w4137, w4129) -> (w4139:bool[])
        n2517 = Compound Arithmetic op=OR("Save Calibration", w4137, w4124, w4129) -> (w4142:bool)
        n2518 = Boolean Array To Number(Boolean array=w4139) -> (number=w4136:u32)
        n2519 = feedback #28(FALSE ("Save APD Data\nwith Trap Data")) -> (w4118:bool)
        n2520 = feedback #29(refnum<k0> refnum) -> (w4145:refnum<file>)
        n2521 = feedback #30(refnum<k0> refnum) -> (w4120:refnum<file>)
        n2522 = feedback #31(FALSE ("Save APD Data\nwith Trap Data")) -> (w4128:bool)
        n2523 = feedback #32(refnum<k0> refnum) -> (w4131:refnum<file>)
        n2524 = feedback #33(0) -> (w4147:i32)
        n2525 = feedback #34() -> (w4135:u32)  [unwired: 1 out]
        n2526 = case shown="True" w4142 {
          tunnel: [w4154 1] -> w4143
          tunnel: w4147 -> [w4156 _]
          tunnel: [w4155 w4174] -> w4144
          tunnel: w4145 -> [w4155 _]
          tunnel: w4141 -> [_ w4194]
          tunnel: w4134 -> [_ w4192]
          tunnel: w4136 -> [_ w4195]
          tunnel: [w4153 w4173] -> w4133
          tunnel: w4135 -> [w4153 _]
          tunnel: [w4152 w4171] -> w4130
          tunnel: w4131 -> [w4152 _]
          tunnel: [w4151 w4170] -> w4127
          tunnel: w4128 -> [w4151 _]
          tunnel: "Start Saving" -> [_ w4168]
          tunnel: w4123 -> [_ w4167]
          tunnel: [w4150 w4158] -> w4116
          tunnel: w4120 -> [w4150 _]
          tunnel: [w4149 w4157] -> w4117
          tunnel: w4118 -> [w4149 _]
          frame False {
            n2527 = Increment(x=w4156) -> (x+1=w4154:i32)
          }
          frame True {
            w4164 = FALSE ("Start Saving")
            w4169 = 9.0  # File Version
            w4177 = FALSE ("prepend array or string size? (T)")
            w4175 = T24."big-endian, network order" ("byte order (0:big-endian, network order)")
            n2528 = local read "BD 1 Frequency 1 (MHz)"() -> (w4191:dbl)
            n2529 = local read "BD 2 Frequency 1 (MHz)"() -> (w4190:dbl)
            n2530 = local read "BD 1 Frequency 2 (MHz)"() -> (w4189:dbl)
            n2531 = local read "BD 2 Frequency 2 (MHz)"() -> (w4188:dbl)
            n2532 = local read "BD 1 Frequency 3 (MHz)"() -> (w4187:dbl)
            n2533 = local read "BD 2 Frequency 3 (MHz)"() -> (w4186:dbl)
            n2534 = Array Size(array=w4167) -> (size(s)=w4166:i32)
            n2535 = To Double Precision Float(number=w4166) -> (double precision float=w4165:dbl)
            n2536 = local write "Save Calibration"(w4164) -> ()
            n2537 = local write "Start Saving"(w4164) -> ()
            n2538 = Build Array("Save APD Data\nwith Trap Data", "Save Trap Pos. Data") -> (w4161:bool[])
            n2539 = Boolean Array To Number(Boolean array=w4161) -> (number=w4160:u32)
            n2540 = Build Array(w4191, w4190, w4189, w4188, w4187, w4186) -> (w4185:dbl[])
            n2541 = case shown="4" w4195 {
              tunnel: w4194 -> [w4266 w4286 w4302 w4340]
              tunnel: w4165 -> [w4271 w4293 w4322 w4359]
              tunnel: w4192 -> [w4270 w4292 w4321 w4358]
              tunnel: [w4267 w4288 w4313 w4350] -> w4183
              tunnel: [w4258 "Cal sets to save" w4303 w4341] -> w4173
              tunnel: w4185 -> [w4268 w4289 w4315 w4352]
              tunnel: "Save APD Data\nwith Trap Data" -> [w4265 _ w4299 w4338]
              tunnel: [w4265 w4280 w4299 w4338] -> w4170
              tunnel: w4169 -> [w4261 w4281 w4297 w4336]
              tunnel: w4168 -> [w4260 _ _ _]
              tunnel: [w4251 w4280 w4296 w4326] -> w4157
              tunnel: "Save Trap Pos. Data" -> [w4251 _ w4296 w4326]
              tunnel: w4160 -> [w4250 _ w4295 w4325]
              frame 1, Default {
                # "timeseries"
                n2542 = case shown="True" "Profile" {
                  tunnel: [w4274 w4278] -> w4255
                  tunnel: [w4274 w4277] -> w4254
                  tunnel: [w4274 w4276] -> w4253
                  tunnel: [w4274 w4275] -> w4252
                  frame False {
                    w4274 = 0.0 ("f")
                  }
                  frame True {
                    n2543 = local read "Current Position"() -> (w4279:cluster{dbl, dbl, dbl})
                    n2544 = local read "Y change (mm)"() -> (w4275:dbl)
                    n2545 = Unbundle(w4279) -> (w4278:dbl, w4277:dbl, w4276:dbl)
                  }
                }
                n2546 = local read "Save ave N"() -> (w4273:dbl)
                n2547 = Multiply(x=w4273, y=w4266) -> (x*y=w4272:dbl)
                n2548 = To Double Precision Float(number=w4250) -> (double precision float=w4264:dbl)
                n2549 = Build Array(w4261, w4266, w4272, w4271, w4270, 0.0 ("f")) -> (w4269:dbl[])
                n2550 = Build Array(w4264, w4255, w4254, w4253, w4252) -> (w4262:dbl[])
                n2551 = Select(t=u32 4000000000, s=w4260, f="N sets to save") -> (s? t:f=w4258:u32)
                n2552 = Build Array (concatenate)(w4269, w4268, w4262) -> (w4267:dbl[])
              }
              frame 2 {
                w4283 = 0.0 ("f")
                w4280 = FALSE ("Save APD Data\nwith Trap Data")
                # "calibration"
                n2553 = Boolean To (0,1)(Boolean=w4280) -> (0, 1=w4285:i16)
                n2554 = To Double Precision Float(number=w4285) -> (double precision float=w4284:dbl)
                n2555 = Build Array(w4284, w4283, w4283, w4283, w4283) -> (w4282:dbl[])
                n2556 = Build Array(w4281, w4286, w4286, w4293, w4292, 1.0 ("t")) -> (w4290:dbl[])
                n2557 = Build Array (concatenate)(w4290, w4289, w4282) -> (w4288:dbl[])
                "Calibrating Trap..." <- TRUE ("Calibrating...")
              }
              frame 4 {
                w4300 = 0.0 ("f")
                # "scan dir (x/y = 0/1)"
                # "cycles/step"
                # "n scans (f/b)"
                # "steps"
                # "freq. range"
                # "AOD raster scan"
                n2558 = local read "Number of F/B Scans (AOD)"() -> (w4307:u16)
                n2559 = local read "Cycles/step (AOD)"() -> (w4309:u64)
                n2560 = local read "Scan Range (MHz)"() -> (w4312:dbl)
                n2561 = local read "Scan steps (AOD)"() -> (w4311:u64)
                n2562 = local read "Scan BD"() -> (w4319:bool)
                n2563 = local read "Save ave N"() -> (w4324:dbl)
                n2564 = Boolean To (0,1)(Boolean=w4319) -> (0, 1=w4318:i16)
                n2565 = To Double Precision Float(number=w4307) -> (double precision float=w4306:dbl)
                n2566 = To Double Precision Float(number=w4311) -> (double precision float=w4310:dbl)
                n2567 = To Double Precision Float(number=w4309) -> (double precision float=w4308:dbl)
                n2568 = To Double Precision Float(number=w4318) -> (double precision float=w4317:dbl)
                n2569 = Multiply(x=w4324, y=w4302) -> (x*y=w4323:dbl)
                n2570 = To Double Precision Float(number=w4295) -> (double precision float=w4301:dbl)
                n2571 = Build Array(w4301, w4300, w4300, w4300, w4300) -> (w4298:dbl[])
                n2572 = local read "N sets should be saved"() -> (w4304:dbl)
                n2573 = Build Array(w4317, w4312, w4310, w4308, w4306) -> (w4314:dbl[])
                n2574 = Build Array(w4297, w4302, w4323, w4322, w4321, 2.0 ("t")) -> (w4316:dbl[])
                n2575 = Round Toward +Infinity(x=w4304) -> (ceil(x): smallest int >= x=w4305:dbl)
                n2576 = Build Array (concatenate)(w4316, w4315, w4298, w4314) -> (w4313:dbl[])
                n2577 = To Unsigned Long Integer(number=w4305) -> (unsigned 32bit integer=w4303:u32)
              }
              frame 8 {
                w4333 = 0.0 ("f")
                # "MCL raster scan"
                n2578 = local read "Number of scans (MCL)"() -> (w4328:u64)
                n2579 = local read "Scan lines (y)"() -> (w4327:u64)
                n2580 = local read "2D or 1D Scan"() -> (w4330:bool)
                n2581 = local read "Scan Range (V)\n(of steps)"() -> (w4349:dbl)
                n2582 = local read "Fast Scan Dir"() -> (w4356:bool)
                n2583 = local read "Cycles/step (MCL)"() -> (w4346:u64)
                n2584 = local read "Scan steps (MCL)"() -> (w4348:u64)
                n2585 = Select(t=w4327, s=w4330, f=w4328) -> (s? t:f=w4329:u64)
                n2586 = Boolean To (0,1)(Boolean=w4330) -> (0, 1=w4332:i16)
                n2587 = local read "Save ave N"() -> (w4361:dbl)
                n2588 = local read "Initial X"() -> (w4335:dbl)
                n2589 = local read "Initial Y"() -> (w4334:dbl)
                n2590 = To Double Precision Float(number=w4332) -> (double precision float=w4331:dbl)
                n2591 = Boolean To (0,1)(Boolean=w4356) -> (0, 1=w4355:i16)
                n2592 = To Double Precision Float(number=w4329) -> (double precision float=w4344:dbl)
                n2593 = To Double Precision Float(number=w4348) -> (double precision float=w4347:dbl)
                n2594 = To Double Precision Float(number=w4346) -> (double precision float=w4345:dbl)
                n2595 = To Double Precision Float(number=w4355) -> (double precision float=w4354:dbl)
                n2596 = Multiply(x=w4361, y=w4340) -> (x*y=w4360:dbl)
                n2597 = To Double Precision Float(number=w4325) -> (double precision float=w4339:dbl)
                n2598 = local read "N sets should be saved (MCL)"() -> (w4342:dbl)
                n2599 = Build Array(w4339, w4331, w4333, w4333, w4333) -> (w4337:dbl[])
                n2600 = Build Array(w4354, w4349, w4347, w4345, w4344, w4335, w4334) -> (w4351:dbl[])
                n2601 = Build Array(w4336, w4340, w4360, w4359, w4358, 3.0 ("t")) -> (w4353:dbl[])
                n2602 = Round Toward +Infinity(x=w4342) -> (ceil(x): smallest int >= x=w4343:dbl)
                n2603 = Build Array (concatenate)(w4353, w4352, w4337, w4351) -> (w4350:dbl[])
                n2604 = To Unsigned Long Integer(number=w4343) -> (unsigned 32bit integer=w4341:u32)
              }
            }
            n2605 = local read "Index"() -> (w4200:dbl)
            n2606 = call "Create new save file.vi"("Insert"="", "Ext"=".dat", "Index In"=w4200) -> ("Path Out"=w4159:path, "Index Out"=w4172:dbl)
            n2607 = local write "Save file name"(w4159) -> ()
            n2608 = local write "Index"(w4172) -> ()
            n2609 = local write "Save index"(w4172) -> ()
            n2610 = Array Size(array=w4183) -> (size(s)=w4184:i32)
            n2611 = Open/Create/Replace File(file path (use dialog)=w4159, operation (0:open)=T25."create", access (0:read/write)=enum16{"read/write", "read-only", "write-only"}."write-only") -> (refnum out=w4197:refnum<file>)  [unwired: 1 in, 4 out]
            n2612 = local write "Saving..."(TRUE ("Saving...")) -> ()
            n2613 = To Double Precision Float(number=w4184) -> (double precision float=w4182:dbl)
            n2614 = String Length(string="Comment (data description)") -> (length=w4180:i32)
            n2615 = To Double Precision Float(number=w4180) -> (double precision float=w4179:dbl)
            n2616 = Deny Access(7:w4197) -> (3:w4196:refnum<file>)  [unwired: 1 in, 2 out]
            n2617 = Build Array (concatenate)(w4182, w4183, w4179) -> (w4181:dbl[])
            n2618 = case "If fluorescence data to be saved" shown="True" w4170 {
              tunnel: w4159 -> [_ w4249]
              tunnel: [refnum<k0> refnum w4229] -> w4171
              frame False {
              }
              frame True {
                w4228 = 0.0
                n2619 = local read "APD Integration Time (s)"() -> (w4234:dbl)
                n2620 = local read "N APD Samp/step"() -> (w4227:dbl)
                n2621 = Path To String(path=w4249) -> (string=w4248:string)
                n2622 = String Length(string=w4248) -> (length=w4247:i32)
                n2623 = Subtract(x=w4247, y=4) -> (x-y=w4245:i32)
                n2624 = String Subset(string=w4248, length (rest)=w4245) -> (substring=w4244:string)  [unwired: 1 out]
                n2625 = Build Array(w4234, w4227, w4228, w4228, w4228, w4228, w4228, w4228) -> (w4231:dbl[])
                n2626 = Concatenate Strings(w4244, "_fl.dat" ("string")) -> (w4242:string)
                n2627 = Array Size(array=w4231) -> (size(s)=w4233:i32)
                n2628 = String To Path(string=w4242) -> (path=w4238:path)
                n2629 = Open/Create/Replace File(file path (use dialog)=w4238, operation (0:open)=T25."create", access (0:read/write)=enum16{"read/write", "read-only", "write-only"}."write-only") -> (refnum out=w4239:refnum<file>)  [unwired: 1 in, 4 out]
                n2630 = Deny Access(7:w4239) -> (3:w4235:refnum<file>)  [unwired: 1 in, 2 out]
                n2631 = To Double Precision Float(number=w4233) -> (double precision float=w4232:dbl)
                n2632 = Build Array (concatenate)(w4232, w4231) -> (w4230:dbl[])
                n2633 = Write to Binary File(file (use dialog)=w4235, data=w4230, 5:FALSE ("prepend array or string size? (T)"), 9:T24."big-endian, network order" ("byte order (0:big-endian, network order)")) -> (refnum out=w4229:refnum<file>)  [unwired: 1 in, 3 out]
              }
            }
            n2634 = case shown="True" w4157 {
              tunnel: w4159 -> [_ w4211]
              tunnel: [refnum<k0> refnum w4210] -> w4158
              frame False {
              }
              frame True {
                w4206 = 0.0 ("element")
                n2635 = Path To String(path=w4211) -> (string=w4225:string)
                n2636 = Build Array(w4206, w4206, w4206, w4206, w4206, w4206, w4206, w4206) -> (w4207:dbl[])
                n2637 = String Length(string=w4225) -> (length=w4224:i32)
                n2638 = Subtract(x=w4224, y=4) -> (x-y=w4222:i32)
                n2639 = Array Size(array=w4207) -> (size(s)=w4209:i32)
                n2640 = String Subset(string=w4225, length (rest)=w4222) -> (substring=w4221:string)  [unwired: 1 out]
                n2641 = To Double Precision Float(number=w4209) -> (double precision float=w4208:dbl)
                n2642 = Concatenate Strings(w4221, "_pos.dat" ("string")) -> (w4219:string)
                n2643 = Build Array (concatenate)(w4208, w4207) -> (w4205:dbl[])
                n2644 = String To Path(string=w4219) -> (path=w4215:path)
                n2645 = Open/Create/Replace File(file path (use dialog)=w4215, operation (0:open)=T25."create", access (0:read/write)=enum16{"read/write", "read-only", "write-only"}."write-only") -> (refnum out=w4216:refnum<file>)  [unwired: 1 in, 4 out]
                n2646 = Deny Access(7:w4216) -> (3:w4212:refnum<file>)  [unwired: 1 in, 2 out]
                n2647 = Write to Binary File(file (use dialog)=w4212, data=w4205, 5:FALSE ("prepend array or string size? (T)"), 9:T24."big-endian, network order" ("byte order (0:big-endian, network order)")) -> (refnum out=w4210:refnum<file>)  [unwired: 1 in, 3 out]
              }
            }
            n2648 = Write to Binary File(file (use dialog)=w4196, data=w4181, 5:w4177, 9:w4175) -> (refnum out=w4178:refnum<file>)  [unwired: 1 in, 3 out]
            n2649 = Write to Binary File(file (use dialog)=w4178, data="Comment (data description)", 5:w4177, 9:w4175) -> (refnum out=w4174:refnum<file>)  [unwired: 1 in, 3 out]
          }
        }
        n2650 = feedback-in #28(w4117) -> ()
        n2651 = feedback-in #29(w4144) -> ()
        n2652 = feedback-in #30(w4116) -> ()
        n2653 = feedback-in #31(w4127) -> ()
        n2654 = feedback-in #32(w4130) -> ()
        n2655 = feedback-in #33(w4143) -> ()
        n2656 = feedback-in #34(w4133) -> ()
      }
      frame #1 {
        n2657 = local read "Saving..."() -> (w4374:bool)
        n2658 = case shown="True" w4374 {
          tunnel: w4378 -> [_ w4388]
          tunnel: w4377 -> [_ w4402]
          tunnel: w4376 -> [_ w4398]
          tunnel: w4375 -> [_ w4397]
          tunnel: w4373 -> [_ w4396]
          tunnel: w4372 -> [_ w4391]
          tunnel: w4371 -> [_ w4390]
          tunnel: w4370 -> [_ w4389]
          tunnel: w4369 -> [_ w4387]
          tunnel: w4368 -> [_ w4385]
          tunnel: w4367 -> [_ w4384]
          tunnel: w4366 -> [_ w4383]
          tunnel: w4365 -> [_ w4382]
          tunnel: w4364 -> [_ w4381]
          tunnel: w4363 -> [_ w4380]
          tunnel: w4362 -> [_ w4379]
          frame False {
          }
          frame True {
            n2659 = Multiply(x=w4388, y=w4387) -> (x*y=→"Time (s)":dbl)
            n2660 = Less Or Equal?(x=w4388, y=w4396) -> (x <= y?=w4400:bool)
            n2661 = Or(x="Stop Saving", y="Abort save 2") -> (x .or. y?=w4392:bool)
            n2662 = Not(x=w4392) -> (.not. x?=w4401:bool)
            n2663 = And(x=w4400, y=w4401) -> (x .and. y?=w4399:bool)
            n2664 = case shown="True" w4399 {
              tunnel: w4402 -> [w4409 w4477]
              tunnel: [0.0 w4480] -> w4395
              tunnel: w4388 -> [_ w4478]
              tunnel: w4396 -> [_ w4479]
              tunnel: w4398 -> [_ w4474]
              tunnel: w4397 -> [_ _]
              tunnel: w4391 -> [w4407 w4467]
              tunnel: w4390 -> [w4406 w4468]
              tunnel: w4389 -> [_ w4466]
              tunnel: w4385 -> [_ w4465]
              tunnel: w4384 -> [_ w4419]
              tunnel: w4383 -> [_ w4458]
              tunnel: w4382 -> [_ w4436]
              tunnel: w4381 -> [w4403 w4417]
              tunnel: w4380 -> [w4404 w4416]
              tunnel: w4379 -> [_ w4413]
              frame False {
                w4405 = FALSE
                n2665 = Close File(refnum=w4409) -> ()  [unwired: 1 in, 2 out]
                n2666 = case shown="True" w4406 {
                  tunnel: w4407 -> [_ w4411]
                  frame False {
                  }
                  frame True {
                    n2667 = Close File(refnum=w4411) -> ()  [unwired: 1 in, 2 out]
                  }
                }
                n2668 = case shown="True" w4403 {
                  tunnel: w4404 -> [_ w4410]
                  frame False {
                  }
                  frame True {
                    n2669 = Close File(refnum=w4410) -> ()  [unwired: 1 in, 2 out]
                  }
                }
                n2670 = local write "Raster Scanning..."(w4405) -> ()
                n2671 = local write "Calibrating Trap..."(w4405) -> ()
                n2672 = call <vilib>:"Beep.vi"() -> ()  [unwired: 3 in, 9 out]
                n2673 = local write "Stop Saving"(w4405) -> ()
                "Saving..." <- w4405
              }
              frame True {
                n2674 = local read "Calibrating Trap..."() -> (w4469:bool)
                n2675 = case "Write fl. data" shown="True" w4468 {
                  tunnel: w4467 -> [_ w4503]
                  tunnel: w4466 -> [_ w4502]
                  frame False {
                  }
                  frame True {
                    n2676 = Write to Binary File(file (use dialog)=w4503, data=w4502, 5:FALSE ("prepend array or string size? (T)"), 9:T24."big-endian, network order" ("byte order (0:big-endian, network order)")) -> ()  [unwired: 1 in, 4 out]
                  }
                }
                n2677 = Greater?(x="Save ave N", y=1.0) -> (0:w4472:bool)
                n2678 = Not(x=w4469) -> (.not. x?=w4471:bool)
                n2679 = And(x=w4471, y=w4472) -> (x .and. y?=w4414:bool)
                n2680 = case shown="True" w4414 {
                  tunnel: w4413 -> [w4483 w4494]
                  tunnel: [w4483 w4486] -> w4412
                  tunnel: "Save ave N" -> [_ w4487]
                  frame False {
                  }
                  frame True {
                    w4484 = 2 ("dimension size")
                    n2681 = Array Size(array=w4494) -> (size(s)=w4488:i32)
                    n2682 = Divide(x=w4488, y=w4484) -> (x/y=w4492:dbl)
                    n2683 = Reshape Array(w4494, w4492, w4484) -> (w4493:u64[][])
                    n2684 = Transpose 2D Array(2D array=w4493) -> (transposed array=w4491:u64[][])
                    n2685 = for {
                      tunnel: w4491 -> [w4496] mode=indexing
                      tunnel: [w4495] -> w4485 mode=indexing
                      tunnel: w4487 -> [w4497]
                      workers-P: _ -> [_]
                      n2686 = call "downsample 1D array - U64.vi"("Ave N"=w4497, "Array In"=w4496) -> ("Array Out"=w4495:u64[])  [unwired: 1 in]
                    }
                    n2687 = Transpose 2D Array(2D array=w4485) -> (transposed array=w4490:u64[][])
                    n2688 = Divide(x=w4488, y=w4487) -> (x/y=w4489:dbl)
                    n2689 = Reshape Array(w4490, w4489) -> (w4486:u64[])
                  }
                }
                n2690 = case shown="False" w4414 {
                  tunnel: w4474 -> [w4506 w4518]
                  tunnel: [w4506 w4510] -> w4470
                  tunnel: "Save ave N" -> [_ w4511]
                  tunnel: w4465 -> [_ w4509]
                  frame False {
                  }
                  frame True {
                    n2691 = Array Size(array=w4518) -> (size(s)=w4512:i32)
                    n2692 = Array Size(array=w4509) -> (size(s)=w4508:i32)
                    n2693 = Divide(x=w4512, y=w4508) -> (x/y=w4516:dbl)
                    n2694 = Reshape Array(w4518, w4516, w4508) -> (w4517:i16[][])
                    n2695 = Transpose 2D Array(2D array=w4517) -> (transposed array=w4515:i16[][])
                    n2696 = for {
                      tunnel: w4515 -> [w4521] mode=indexing
                      tunnel: [w4520] -> w4507 mode=indexing
                      tunnel: w4511 -> [w4519]
                      workers-P: _ -> [_]
                      n2697 = call "downsample 1D array - I16.vi"("Ave N"=w4519, "Array In"=w4521) -> ("Array Out"=w4520:i16[])  [unwired: 1 out]
                    }
                    n2698 = Transpose 2D Array(2D array=w4507) -> (transposed array=w4514:i16[][])
                    n2699 = Divide(x=w4512, y=w4511) -> (x/y=w4513:dbl)
                    n2700 = Reshape Array(w4514, w4513) -> (w4510:i16[])
                  }
                }
                n2701 = Index Array(array=w4436, index=1) -> (element=w4439:waveform(dbl))
                n2702 = Index Array(array=w4436, index=0) -> (element=w4441:waveform(dbl))
                n2703 = Unbundle By Name(w4439) -> ("Y"=w4443:dbl[])
                n2704 = Unbundle By Name(w4441) -> ("Y"=w4451:dbl[])
                n2705 = case "Write trap pos. data" shown="True" w4417 {
                  tunnel: w4416 -> [_ w4499]
                  tunnel: w4412 -> [_ w4498]
                  frame False {
                  }
                  frame True {
                    n2706 = Write to Binary File(file (use dialog)=w4499, data=w4498, 5:FALSE ("prepend array or string size? (T)"), 9:T24."big-endian, network order" ("byte order (0:big-endian, network order)")) -> ()  [unwired: 1 in, 4 out]
                  }
                }
                n2707 = Write to Binary File(file (use dialog)=w4477, data=w4470, 5:FALSE ("prepend array or string size? (T)"), 9:T24."big-endian, network order" ("byte order (0:big-endian, network order)")) -> ()  [unwired: 1 in, 4 out]
                n2708 = feedback #35(w4443) -> (w4445:dbl[])
                n2709 = Build Array (concatenate)(w4445, w4443) -> (w4444:dbl[])
                n2710 = Select(t=w4443, s=w4419, f=w4444) -> (s? t:f=w4429:dbl[])
                n2711 = feedback-in #35(w4429) -> ()
                n2712 = feedback #36(w4451) -> (w4464:dbl[])
                n2713 = Build Array (concatenate)(w4464, w4451) -> (w4463:dbl[])
                n2714 = Select(t=w4451, s=w4419, f=w4463) -> (s? t:f=w4438:dbl[])
                n2715 = feedback-in #36(w4438) -> ()
                n2716 = Divide(x=w4478, y=w4479) -> (x/y=w4481:dbl)
                n2717 = Multiply(x=w4481, y=100.0) -> (x*y=w4480:dbl)
                n2718 = Build Array(w4438, w4429) -> (→"Saved APD":dbl[][])
                n2719 = Array Size(array=w4438) -> (size(s)=w4456:i32)
                n2720 = Unbundle By Name(w4458) -> ("Y"=w4462:dbl[])
                n2721 = Subtract(x=w4456, y="N pts to average") -> (x-y=w4432:i32)
                n2722 = Multiply(x="N pts to average", y=u16 2) -> (x*y=w4433:u16)
                n2723 = Subtract(x=w4456, y=w4433) -> (x-y=w4431:i32)
                n2724 = feedback #37(w4462) -> (w4461:dbl[])
                n2725 = Build Array (concatenate)(w4461, w4462) -> (w4460:dbl[])
                n2726 = Select(t=w4462, s=w4419, f=w4460) -> (s? t:f=w4459:dbl[])
                "Trap Delta Graph" <- w4459
                n2727 = feedback-in #37(w4459) -> ()
                n2728 = Array Subset(array=w4438, index=w4432, length="N pts to average") -> (w4455:dbl[])
                n2729 = Array Subset(array=w4438, index=w4431, length="N pts to average") -> (w4454:dbl[])
                n2730 = Array Subset(array=w4429, index=w4432, length="N pts to average") -> (w4435:dbl[])
                n2731 = Array Subset(array=w4429, index=w4431, length="N pts to average") -> (w4434:dbl[])
                n2732 = call <vilib>:"Mean.vi"("X"=w4455) -> ("mean"=w4453:dbl)  [unwired: 1 out]
                n2733 = call <vilib>:"Mean.vi"("X"=w4435) -> ("mean"=w4428:dbl)  [unwired: 1 out]
                n2734 = call <vilib>:"Mean.vi"("X"=w4454) -> ("mean"=w4452:dbl)  [unwired: 1 out]
                n2735 = call <vilib>:"Mean.vi"("X"=w4434) -> ("mean"=w4427:dbl)  [unwired: 1 out]
                n2736 = Subtract(x=w4428, y=w4427) -> (x-y=w4418:dbl)
                "Delta Fl. 2" <- w4418
                n2737 = Subtract(x=w4453, y=w4452) -> (x-y=w4450:dbl)
                "Delta Fl. 1" <- w4450
                n2738 = Initialize Array(w4450, 1 ("dimension size")) -> (w4447:dbl[])
                n2739 = Initialize Array(w4418, 1 ("dimension size")) -> (w4424:dbl[])
                n2740 = feedback #38(w4447) -> (w4448:dbl[])
                n2741 = Build Array (concatenate)(w4448, w4447) -> (w4446:dbl[])
                n2742 = feedback #39(w4424) -> (w4425:dbl[])
                n2743 = Build Array (concatenate)(w4425, w4424) -> (w4423:dbl[])
                n2744 = Select(t=w4447, s=w4419, f=w4446) -> (s? t:f=w4422:dbl[])
                n2745 = feedback-in #38(w4422) -> ()
                n2746 = Select(t=w4424, s=w4419, f=w4423) -> (s? t:f=w4421:dbl[])
                n2747 = feedback-in #39(w4421) -> ()
                n2748 = Build Array(w4422, w4421) -> (→"Save APD Deriv":dbl[][])
              }
            }
            "Progress" <- w4395
            "Progress 2" <- w4395
          }
        }
      }
    }
    n2749 = Bundle By Name(cluster=w3057, "Green FB Ch 0"=w3056, "Green FB Ch 1"=w3055) -> (w3035:T47)
    "Green FB Signals (V)" <- w3035
    n2750 = Unbundle By Name(w3035) -> ("Green FB Ch 2"=→"Green FB Plot":dbl)
    n2751 = local read "wait to reset values"() -> (w3126:bool)
    n2752 = Not(x=w3124) -> (.not. x?=w3127:bool)
    n2753 = And(x=w3127, y=w3126) -> (x .and. y?=w3128:bool)
    n2754 = case "Part of MCL raster scanning: returns to initial positions after scan done" shown="True" w3128 {
      tunnel: w2841 -> [w3937 w3944]
      tunnel: [w3937 w3943] -> w3130
      tunnel: w2840 -> [w3936 w3942]
      tunnel: [w3936 w3941] -> w3125
      frame False {
      }
      frame True {
        w3952 = 10.0 ("y")
